vi "Vision Research Phantom Series PhFile PhNewCineFromFile.vi"(2 "szFileName":path, 5 "Error In (no error)":errorcluster) -> (15 "pCH":u64, 19 "Error Out":errorcluster)   [LabVIEW 2013, in "VRI.lvlib"]
doc: "PhFile.dll\n\nPhNewCineFromFile\nHRESULT PhNewCineFromFile(PSTR szFN, PCINEHANDLE pCH);\n\nParameters Description\nszFN(in) Cine file name.\npCH(out) Pointer to handle of the file cine.\nReturn HRESULT (0 = Ok)\nComments This function creates a cine handle that corresponds to a cine file.\n\nWritten by:\nBLOOMY CONTROLS, INC\nWINDSOR, CT 06095, USA\n860-298-9925\nwww.bloomy.com\nV1.0.0\nMay, 2004"
uses:
  VRI.lvlib
  Phantom DLLs/PhFile.dll
panel:
  # "For instructions on the use of this VI, press Ctrl+H to display the help window and move the mouse over the icon, controls, and indicators"
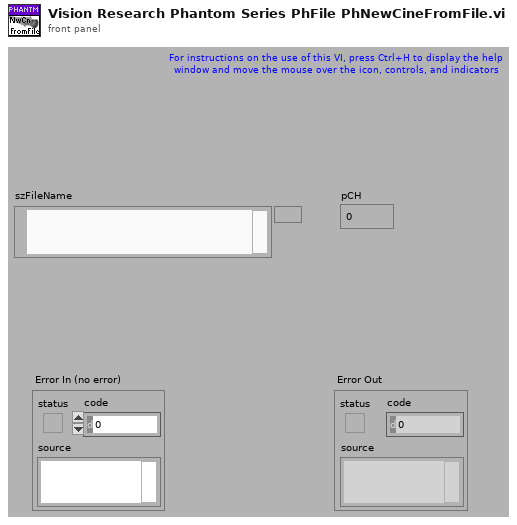
[diagram p1: front panel]
types:
  T1 = enum32{"existing file", "new file", "new or existing file", "existing dir", "new dir", "new or existing dir", "existing file (use LLBs)", "new file (use LLBs)", "new or existing file (use LLBs)", "new or existing file or directory (use LLBs)"}
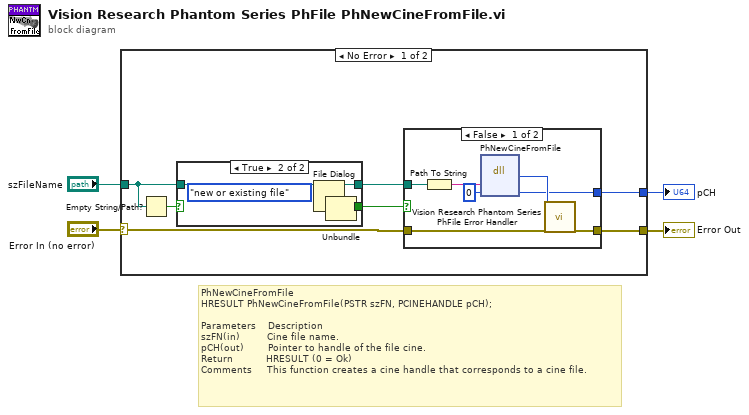
[diagram p0: block diagram]
diagram:
  # "PhNewCineFromFile\nHRESULT PhNewCineFromFile(PSTR szFN, PCINEHANDLE pCH);\n\nParameters    Description\nszFN(in)         Cine file name.\npCH(out)        Pointer to handle of the file cine.\nReturn           HRESULT (0 = Ok)\nComments     This function creates a cine handle that corresponds to a cine file."
  n1 = case shown="No Error" "Error In (no error)" {
    selector: "Error In (no error)" -> [w11 w26]
    tunnel: [w10 w26] -> w3
    tunnel: [w9 _] -> w2
    tunnel: "szFileName" -> [w6 _]
    frame No Error {
      n2 = Empty String/Path?(string/path=w6) -> (empty?=w8:bool)
      n3 = case shown="True" w8 {
        selector: w8 -> [w20 _]
        tunnel: [w21 w24] -> w7
        tunnel: w6 -> [w21 w25]
        tunnel: [w20 w23] -> w5
        frame False {
        }
        frame True {
          (unwired) T1."new or existing file" ("select mode (2)")
          n4 = File Dialog(11:w25) -> (0:w22:errorcluster, 1:w23:bool, 3:w24:path)  [unwired: 1 in, 6 out]
          n5 = Unbundle(w22) -> ()  [unwired: 3 out]
        }
      }
      n6 = case shown="False" w5 {
        tunnel: [w18 w19] -> w10
        tunnel: w11 -> [w17 w19]
        tunnel: w7 -> [w16 _]
        tunnel: [w13 _] -> w9
        frame False {
          n7 = Path To String(path=w16) -> (string=w12:string)
          n8 = dll-call lib="C:/Projects/SDK/32-bit/Vision Research Phantom Series Labview Driver/Phantom DLLs/PhFile.dll" fn="PhNewCineFromFile"("szFN"=w12, "pCH"=u64 0) -> ("HRESULT"=w15:i32, "pCH"=w13:u64)  [unwired: 4 in, 2 out]
          n9 = call "Vision Research Phantom Series PhFile Error Handler.vi"("Error Code (0)"=w15, "Error In (no error)"=w17) -> ("Error Out"=w18:errorcluster)  [unwired: 17 out]
        }
        frame True {
        }
      }
    }
    frame Error {
    }
  }
  "Error Out" <- w3
  "pCH" <- w2
